vi "MiniProject.vi"() -> ()   [LabVIEW 2015]
uses:
  <vilib>/MakerHub/LINX/Public/Peripherals/Analog/Analog Read N Chans.vi
  <vilib>/MakerHub/LINX/Private/Local IO/LinxAnalogRead.vi
  <vilib>/MakerHub/LINX/Public/Utilities/Check Channel.vi
  <vilib>/MakerHub/LINX/Public/Utilities/Open Serial.vi
  <vilib>/MakerHub/LINX/Private/Utilties/Generate Error.vi
  <vilib>/MakerHub/LINX/LMH-LINX.lvlib
panel:
  out "Loop Execution Time (msec)":u32
  out "High SNR signal":dbl(graph)
  out "MIC 2":dbl(graph)
  out "MIC 1":dbl(graph)
  out "MIC 0":dbl(graph)
  in  "Serial Port":refnum<visa-resource-name>="N/A"
  in  "AI Channel(s)":u8[](array[numeric])=[0, 1, 2]
  in  "stop":bool
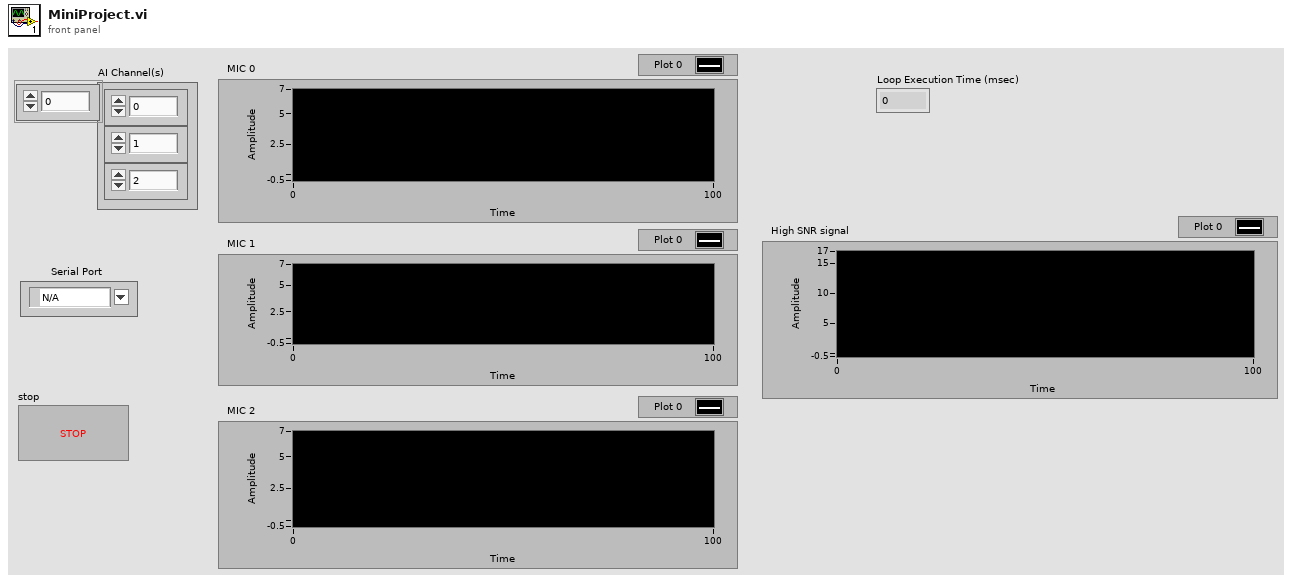
[diagram p1: front panel]
types:
  T1 = typedef "LMH-LINX.lvlib/LINX Ref.ctl" = cluster{"IO":T2, "Interface":T3, "LINX Device Config":T4}
  T2 = typedef "LMH-LINX.lvlib/Platform.ctl" = enum16{"Remote", "Local"}
  T3 = typedef "LMH-LINX.lvlib/Interface.ctl" = enum16{"Serial", "TCP"}
  T4 = typedef "LMH-LINX.lvlib/Device.lvlib/LINX Device Config.ctl" = cluster{"Interface":T3, "COM Port":refnum<visa-resource-name>, "TCP Configuration":T5, "Device Family":u8, "Device ID":u8, "Device Name":string, "TCP Ref":refnum<k5>, "Channels":T6}
  T5 = typedef "LMH-LINX.lvlib/Device.lvlib/TCP Config.ctl" = cluster{"IP Address":string, "Port":u16}
  T6 = typedef "LMH-LINX.lvlib/Channels.ctl" = cluster{"DI":u8[], "DO":u8[], "AI":u8[], "AO":u8[], "PWM":u8[], "QE":u8[], "UART":u8[], "I2C 2":u8[], "SPI":u8[], "CAN":u8[], "Servo":u8[], "AI Ref (V)":dbl, "AI Resolution (Bits)":u8, "AO Ref (V)":dbl, "AO Resolution (Bits)":u8}
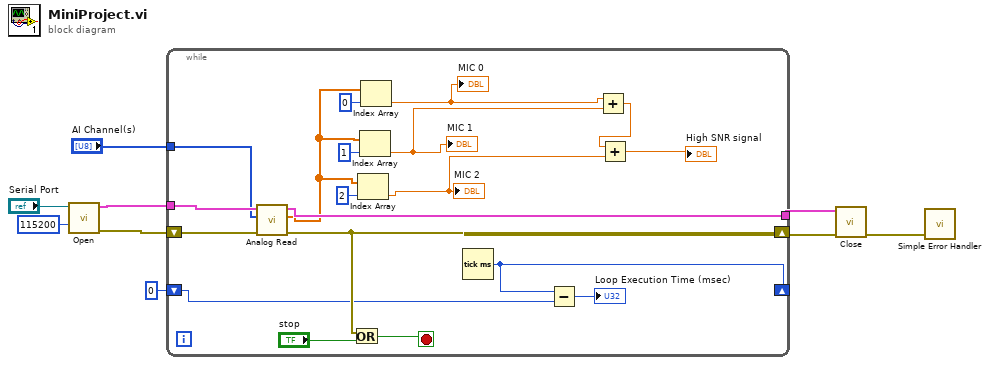
[diagram p0: block diagram]
diagram:
  n1 = call-poly <vilib>:"Open.vi"("Baud Rate Override"=u32 115200, "Serial Port"="Serial Port") -> ("Error Out"=w8:errorcluster, "LINX Resource"=w9:T1)  [unwired: 7 in, 1 out]
  n2 = while {
    shift-right: [w24] -> w7
    shift-left: w8 -> [w27]
    tunnel: w9 -> [w28]
    tunnel: [w26] -> w5
    tunnel: "AI Channel(s)" -> [w22]
    shift-right: [w12] -> _
    shift-left: u32 0 ("millisecond timer value") -> [w11]
    stop <- w23 stop-if-true
    n3 = call-poly <vilib>:"Analog Read.vi"("Error In"=w27, "AI Channel(s)"=w22, "LINX Resource"=w28) -> ("Error Out"=w24:errorcluster, "Voltages"=w18:dbl[], "LINX Resource"=w26:T1)  [unwired: 5 in, 1 out]
    n4 = Or(x=w24, y="stop") -> (x .or. y?=w23:bool)
    n5 = Index Array(array=w18, index=2) -> (element=w15:dbl)
    "MIC 2" <- w15
    n6 = Index Array(array=w18, index=1) -> (element=w14:dbl)
    "MIC 1" <- w14
    n7 = Index Array(array=w18, index=0) -> (element=w16:dbl)
    "MIC 0" <- w16
    n8 = Tick Count (ms)() -> (millisecond timer value=w12:u32)
    n9 = Subtract(x=w12, y=w11) -> (x-y=→"Loop Execution Time (msec)":u32)
    n10 = Add(x=w16, y=w14) -> (x+y=w17:dbl)
    n11 = Add(x=w17, y=w15) -> (x+y=→"High SNR signal":dbl)
  }
  n12 = call <vilib>:"Close.vi"("Error In"=w7, "LINX Resource"=w5) -> ("Error Out"=w6:errorcluster)  [unwired: 9 in]
  n13 = call <vilib>:"Simple Error Handler.vi"("error in (no error)"=w6) -> ()  [unwired: 4 in, 5 out]
